vi "Send Interface Status.vi"(8 "error in (no error)":errorcluster, 10 "Message":string, 11 "RxTx in":refnum<class "RxTx.lvclass">) -> (0 "error out":errorcluster, 3 "RxTx out":refnum<class "RxTx.lvclass">)   [LabVIEW 2018, in "RxTx.lvclass"]
uses:
  RxTx.lvclass
  Interface/Interface.lvclass
  <vilib>/Utility/Data Type/NI_Data Type.lvlib
panel:
  out "Camera Status":T1
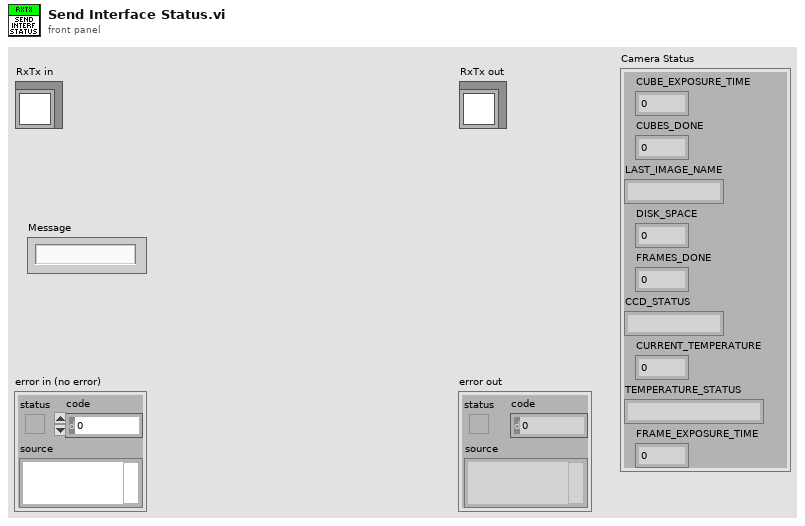
[diagram p1: front panel]
types:
  T1 = cluster{"CUBE_EXPOSURE_TIME":sgl, "CUBES_DONE":u16, "LAST_IMAGE_NAME":string, "DISK_SPACE":u16, "FRAMES_DONE":u16, "CCD_STATUS":string, "CURRENT_TEMPERATURE":i16, "TEMPERATURE_STATUS":string, "FRAME_EXPOSURE_TIME":u16}
  T2 = cluster{"Current Temperature":i16, "Temperatue Status":string}
  T3 = cluster{"Initialization":bool, "Serial Number":u16}
  T4 = cluster{"Exposure Time":sgl, "Pre-amp gain":u8, "Readout Rate":u8, "EM Mode":u8, "EM Gain":u16, "Binning":u16, "Initial Line":u16, "Initial Cloumn":u16, "Final Line":u16, "Final Column":u16, "Kinetic Series Length":u32, "Shutter Mode":u8, "Cooler ON/OFF":u16, "Temperature":i8, "Image Name":string, "Image Path":string, "Cubes":u32, "Trigger":u16}
  T5 = typedef "NI_Data Type.lvlib/Data Type.ctl" = enum8{"Invalid Type", "Void", "I8", "I16", "I32", "I64", "U8", "U16", "U32", "U64", "Single Float", "Double Float", "Extended Float", "Single Complex", "Double Complex", "Extended Complex", "Enum U8", "Enum U16", "Enum U32", "Enum U64", "Single Float With Unit", "Double Float With Unit", "Extended Float With Unit", "Single Complex with Unit", "Double Complex with Unit", "Extended Complex with Unit", "Boolean", "String", "Path", "Picture", "Tag", "Array", "Cluster", "Variant", "LV Variant", "Waveform", "Timestamp", "Digital Waveform", "Digital Data", "ExpressData", "Refnum", "External Data", "VI", "Poly VI", "LabVIEW Class Instance", "Fixed Point"}
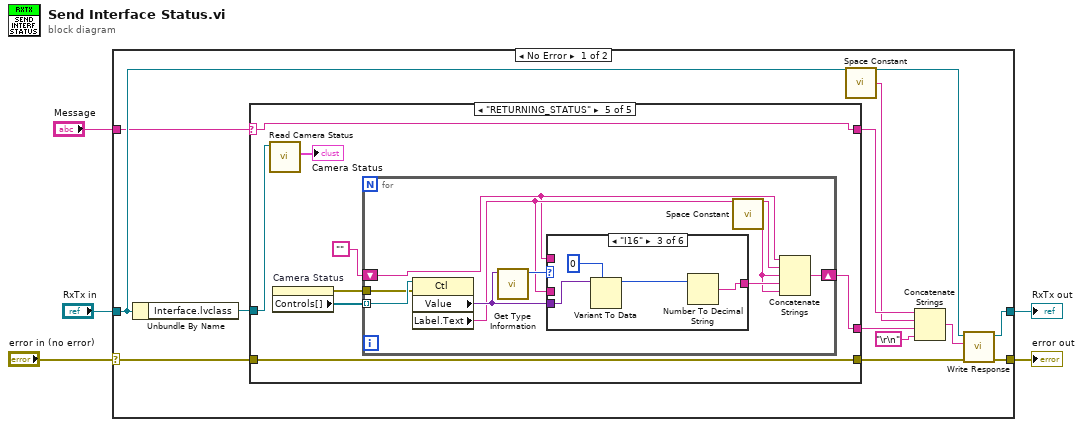
[diagram p0: block diagram]
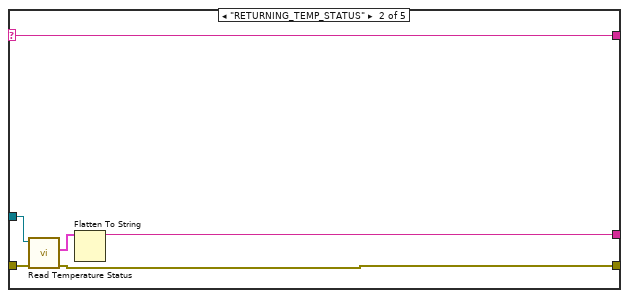
[diagram p3: hidden frame]
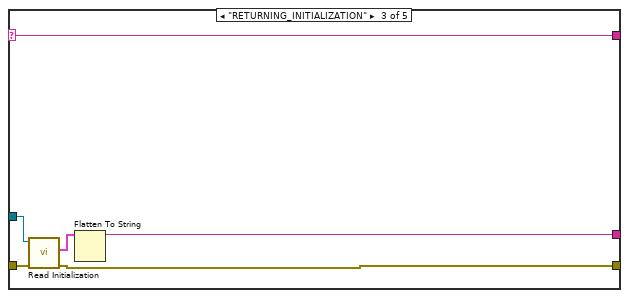
[diagram p4: hidden frame]
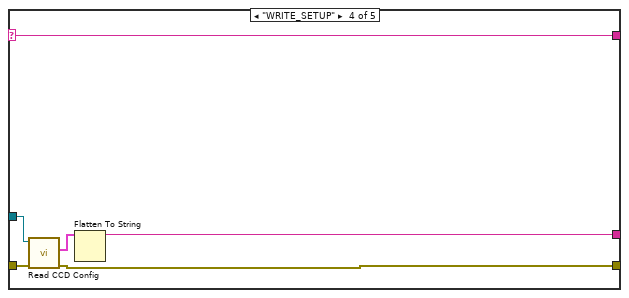
[diagram p5: hidden frame]
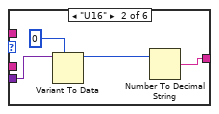
[diagram p7: hidden frame]
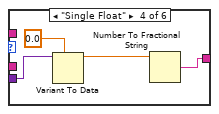
[diagram p8: hidden frame]
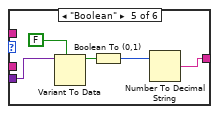
[diagram p9: hidden frame]
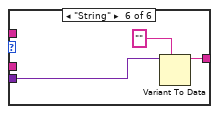
[diagram p10: hidden frame]
diagram:
  n1 = case shown="No Error" "error in (no error)" {
    selector: "error in (no error)" -> [w16 w76]
    tunnel: [w9 w76] -> w2
    tunnel: [w10 w75] -> w1
    tunnel: "RxTx in" -> [w12 w75]
    tunnel: "Message" -> [w6 _]
    frame No Error {
      n2 = Unbundle By Name(w12) -> ("Interface.lvclass"=w17:refnum<class "Interface.lvclass">)
      n3 = case shown="\"RETURNING_STATUS\"" w6 {
        selector: w6 -> [w18 w20 w26 w32 w45]
        tunnel: w17 -> [_ w25 w31 w34 w44]
        tunnel: [w19 w24 w30 w35 w42] -> w14
        tunnel: w16 -> [w19 w23 w29 w36 w42]
        tunnel: [_ w21 w27 w37 w43] -> w15
        tunnel: [w18 w20 w26 w32 w45] -> w11
        frame "False", Default {
        }
        frame "RETURNING_TEMP_STATUS" {
          n4 = call "Read Temperature Status.vi"("error in (no error)"=w23, "Interface in"=w25) -> ("error out"=w24:errorcluster, "Temperature Status"=w22:T2)  [unwired: 7 in, 1 out]
          n5 = Flatten To String(anything=w22) -> (data string=w21:string)  [unwired: 3 in, 2 out]
        }
        frame "RETURNING_INITIALIZATION" {
          n6 = call "Read Initialization.vi"("error in (no error)"=w29, "Interface in"=w31) -> ("error out"=w30:errorcluster, "Initialization"=w28:T3)  [unwired: 7 in, 1 out]
          n7 = Flatten To String(anything=w28) -> (data string=w27:string)  [unwired: 3 in, 2 out]
        }
        frame "WRITE_SETUP" {
          n8 = call "Read CCD Config.vi"("error in (no error)"=w36, "Interface in"=w34) -> ("error out"=w35:errorcluster, "CCD Config"=w33:T4)  [unwired: 7 in, 1 out]
          n9 = Flatten To String(anything=w33) -> (data string=w37:string)  [unwired: 3 in, 2 out]
        }
        frame "RETURNING_STATUS" {
          n10 = call "Read Camera Status.vi"("Interface in"=w44) -> ("Camera Status"=→"Camera Status":T1)  [unwired: 8 in, 2 out]
          n11 = property on="Camera Status" class="Clust (strict)"() -> (error out=w38:errorcluster, "Controls[]"=w39:refnum<vi>[])  [unwired: 2 in, 1 out]
          n12 = for {
            shift-right: [w49] -> w43
            shift-left: "" -> [w51]
            tunnel: w39 -> [w47] mode=indexing
            tunnel: w38 -> [w46]
            n13 = property class="Ctl"(reference=w47, error in=w46) -> ("Value"=w53:variant, "Label.Text"=w52:string)  [unwired: 2 out]
            n14 = call <vilib>:"Get Type Information.vi"("Variant"=w53) -> ("Type"=w54:T5)  [unwired: 6 in, 4 out]
            n15 = case shown="\"I16\"" w54 {
              tunnel: w53 -> [_ w58 w62 w66 w71 w73]
              tunnel: w52 -> [_ _ _ _ _ _]
              tunnel: w51 -> [_ _ _ _ _ _]
              tunnel: [_ w55 w59 w63 w67 w72] -> w50
              frame "Invalid Type", Default {
              }
              frame "U16" {
                n16 = Variant To Data(type=u16 0, Variant=w58) -> (data=w56:u16)  [unwired: 1 in, 1 out]
                n17 = Number To Decimal String(number=w56) -> (decimal integer string=w55:string)  [unwired: 1 in]
              }
              frame "I16" {
                n18 = Variant To Data(type=i16 0, Variant=w62) -> (data=w60:i16)  [unwired: 1 in, 1 out]
                n19 = Number To Decimal String(number=w60) -> (decimal integer string=w59:string)  [unwired: 1 in]
              }
              frame "Single Float" {
                n20 = Variant To Data(type=sgl 0.0, Variant=w66) -> (data=w64:sgl)  [unwired: 1 in, 1 out]
                n21 = Number To Fractional String(number=w64) -> (F-format string=w63:string)  [unwired: 3 in]
              }
              frame "Boolean" {
                n22 = Variant To Data(type=FALSE, Variant=w71) -> (data=w69:bool)  [unwired: 1 in, 1 out]
                n23 = Boolean To (0,1)(Boolean=w69) -> (0, 1=w68:i16)
                n24 = Number To Decimal String(number=w68) -> (decimal integer string=w67:string)  [unwired: 1 in]
              }
              frame "String" {
                n25 = Variant To Data(type="", Variant=w73) -> (data=w72:string)  [unwired: 1 in, 1 out]
              }
            }
            n26 = call <vilib>:"Space Constant.vi"() -> ("String"=w48:string)
            n27 = Concatenate Strings(w51, w52, w48, w50, w48) -> (w49:string)
          }
        }
      }
      n28 = call <vilib>:"Space Constant.vi"() -> ("String"=w7:string)
      n29 = Concatenate Strings(w11, w7, w15, "\r\n") -> (w13:string)
      n30 = call "Write Response.vi"("error in (no error)"=w14, "Response"=w13, "RxTx in"=w12) -> ("error out"=w9:errorcluster, "RxTx out"=w10:refnum<class "RxTx.lvclass">)  [unwired: 7 in]
    }
    frame Error {
    }
  }
  "error out" <- w2
  "RxTx out" <- w1
